vi "Local Setup Config.vi"(0 "KeyName":string, 1 "Local Setup Param":T1, 2 "Config File Directory":path, 5 "KeyValue":string, 9 "Last VI":string, 11 "error in":errorcluster) -> (6 "KeyValues":string[](array[string]), 8 "KeyNames":string[](array[string]), 10 "LastVIs":string[](array[string]), 15 "error out":errorcluster)   [LabVIEW 2014, in "Raspberry Pi Compatible Compiler for LabVIEW.lvlib"]
doc: "Functional Global for reading/writing configuration settings."
uses:
  Raspberry Pi Compatible Compiler for LabVIEW.lvlib
  Custom Controls/Local Setup Parameters.ctl
  <vilib>/Utility/config.llb/Write Key (String).vi
  <vilib>/Utility/config.llb/Read Key (String).vi
  <vilib>/Utility/config.llb/NI_LVConfig.lvlib
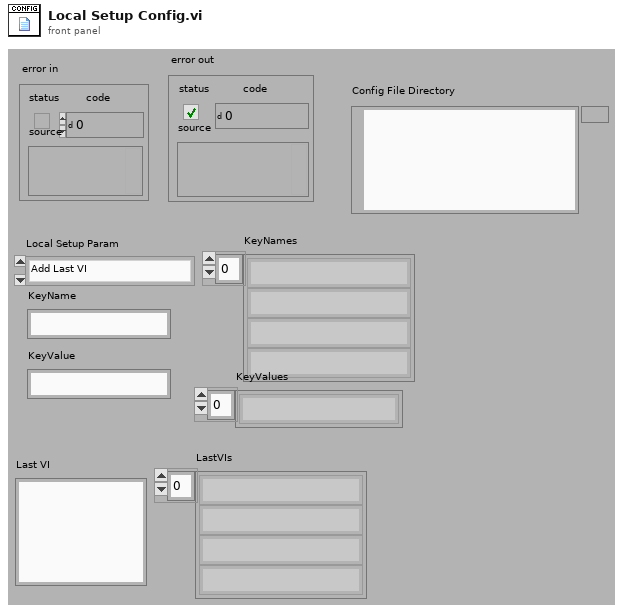
[diagram p1: front panel]
types:
  T1 = typedef "Raspberry Pi Compatible Compiler for LabVIEW.lvlib/Local Setup Parameters.ctl" = enum16{"Add Last VI", "Read Last VI", "Add Board IP", "Remove Board IP", "Read All Board IP", "Add Runtime Version", "Read Runtime Version", "Add Package Version", "Read Package Version", "Add VIPCheck Time", "Read VIPCheck Time"}
  T2 = typedef "NI_LVConfig.lvlib/Config Data RefNum.ctl" = refnum<k1>
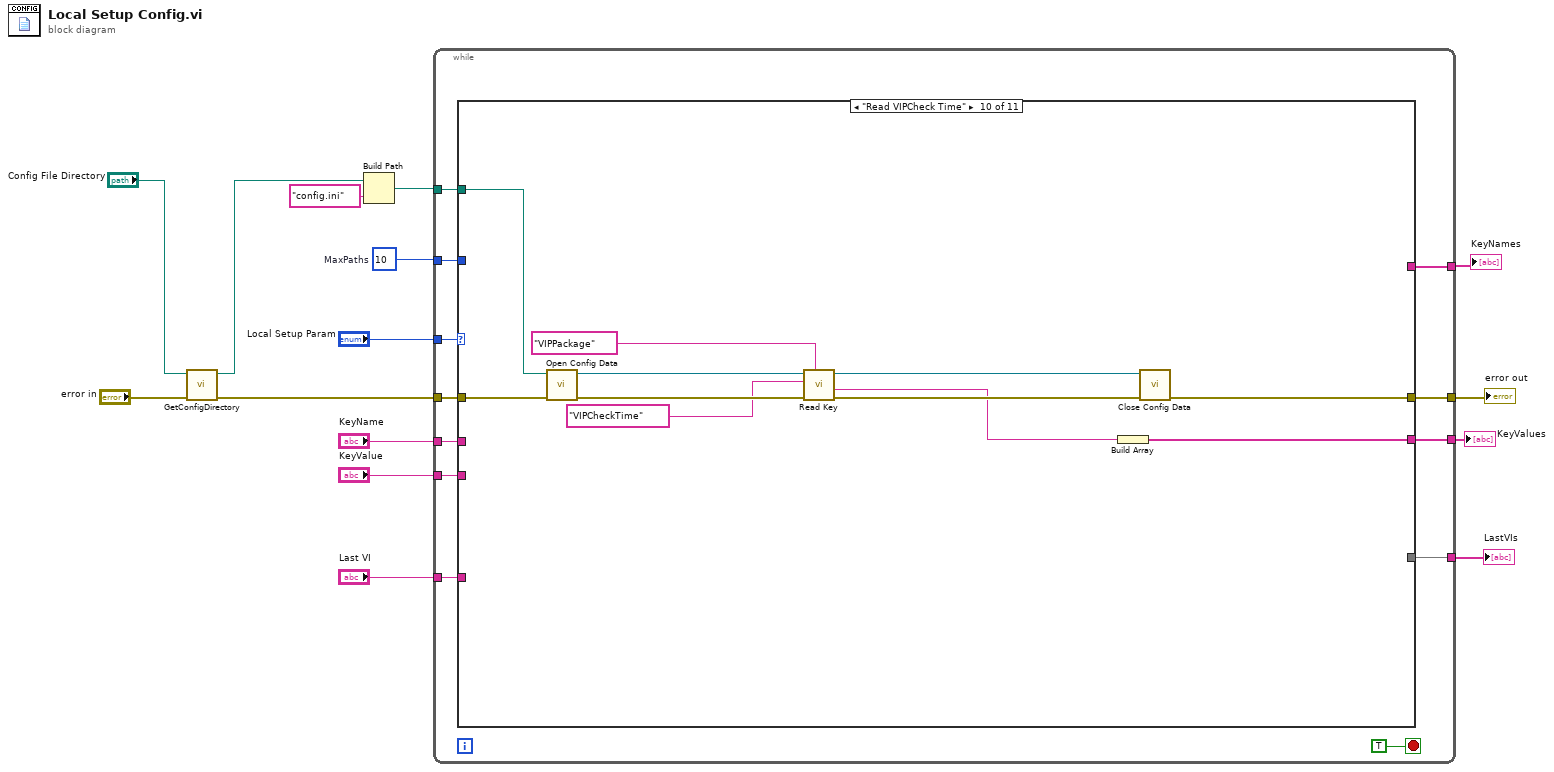
[diagram p0: block diagram]
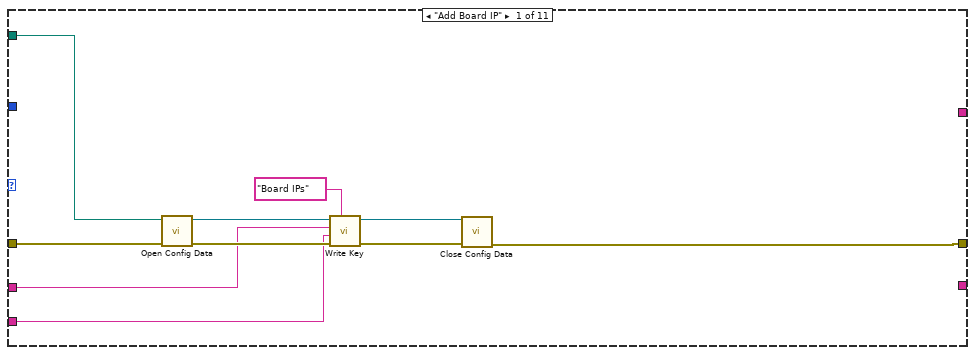
[diagram p2: hidden frame]
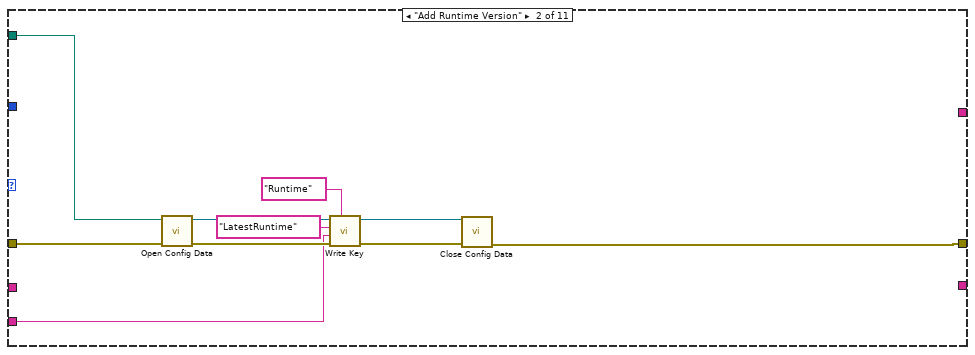
[diagram p3: hidden frame]
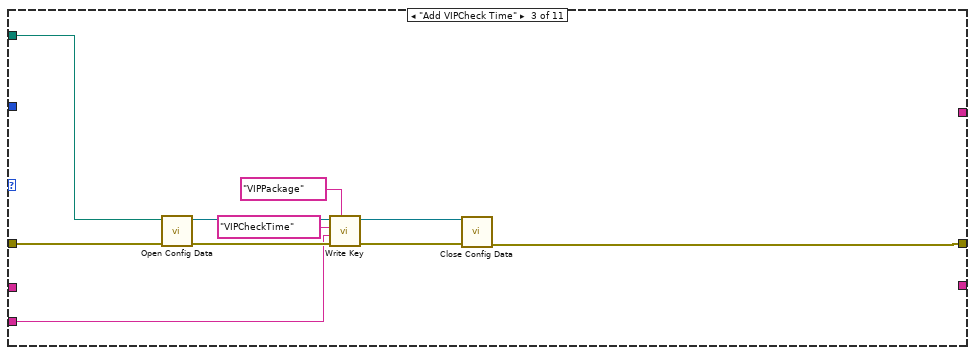
[diagram p4: hidden frame]
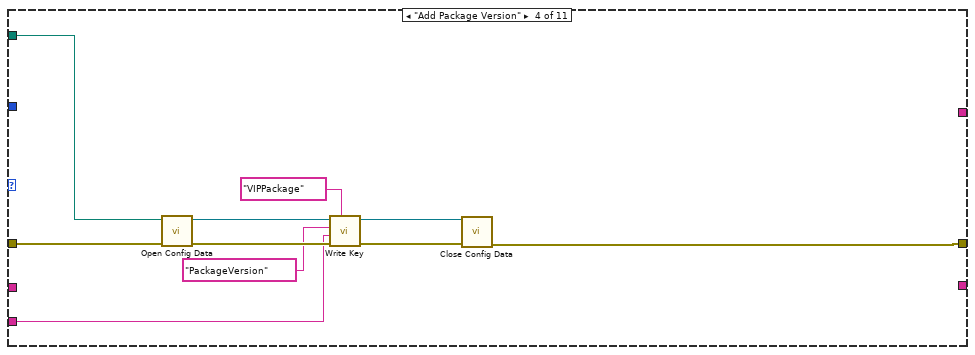
[diagram p5: hidden frame]
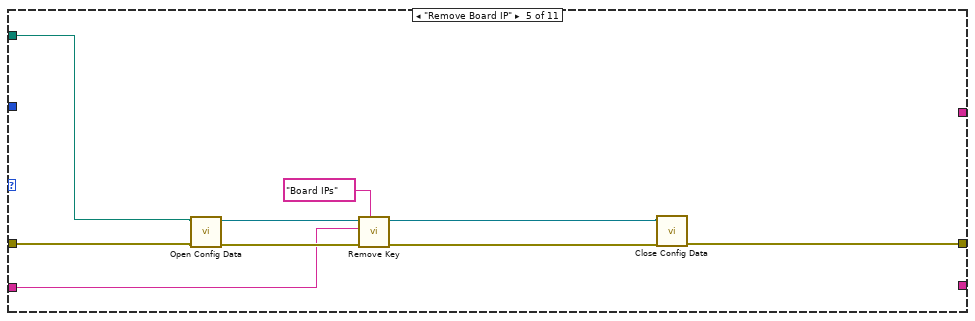
[diagram p6: hidden frame]
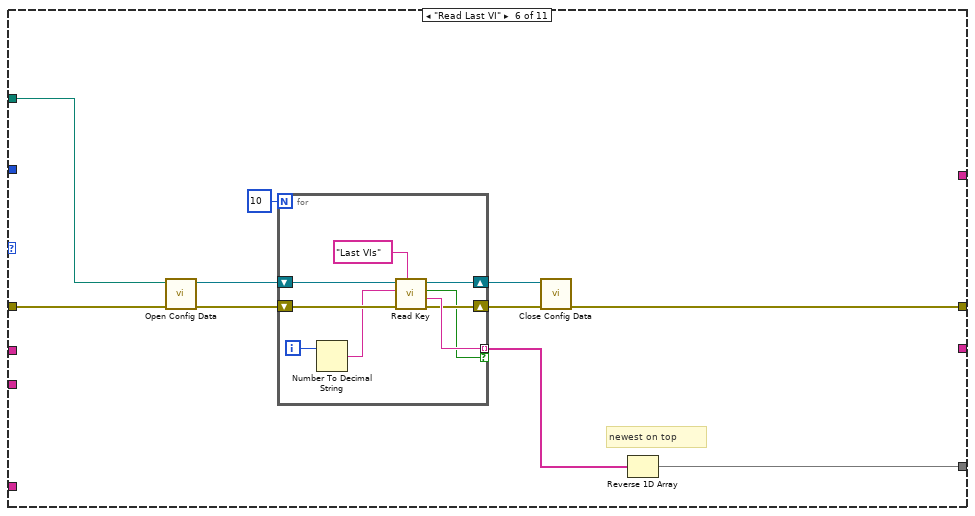
[diagram p7: hidden frame]
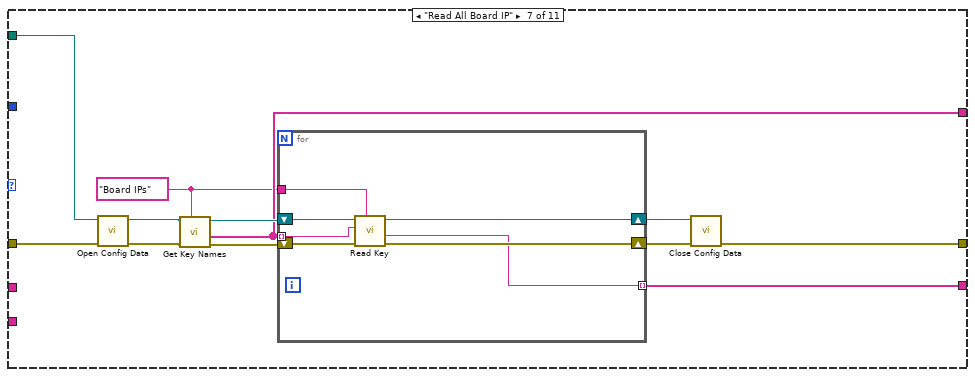
[diagram p8: hidden frame]
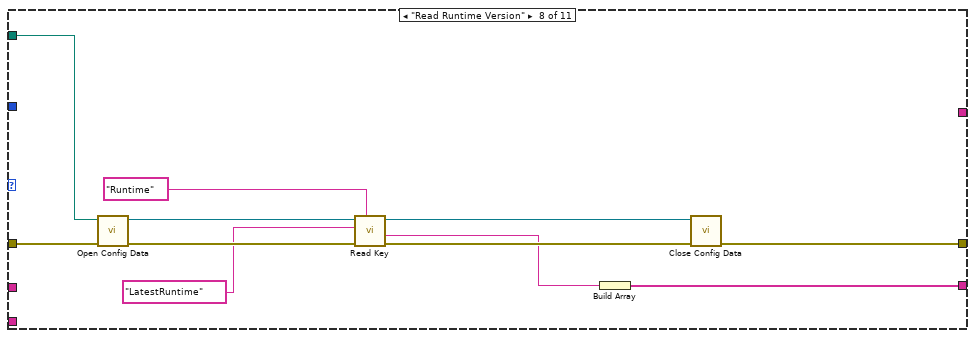
[diagram p9: hidden frame]
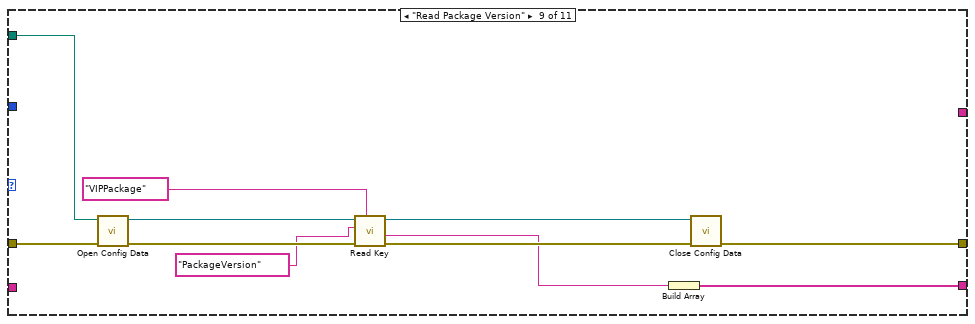
[diagram p10: hidden frame]
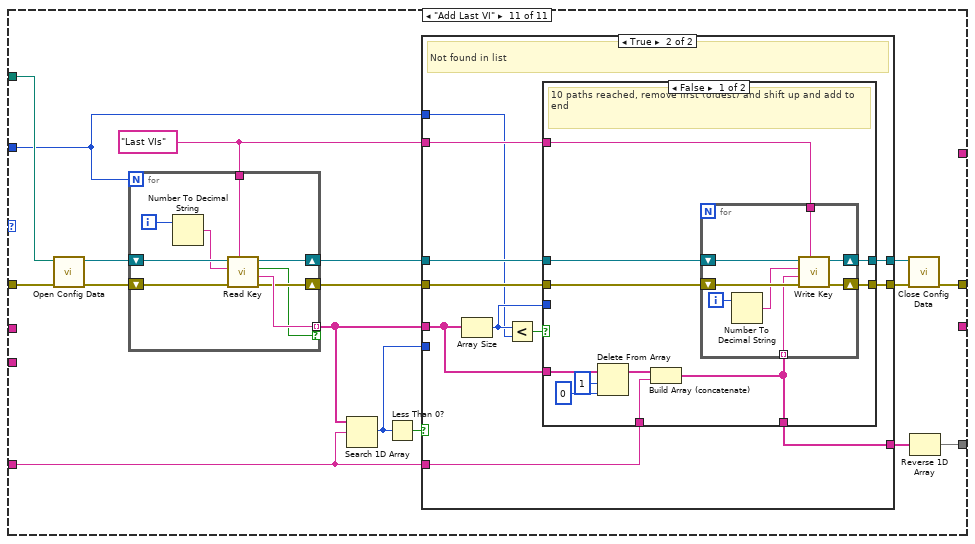
[diagram p11: hidden frame]
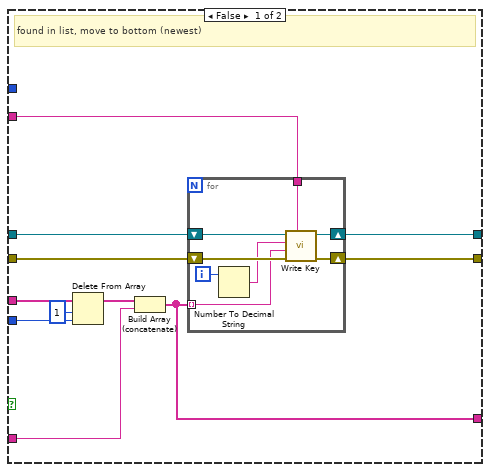
[diagram p12: hidden frame]
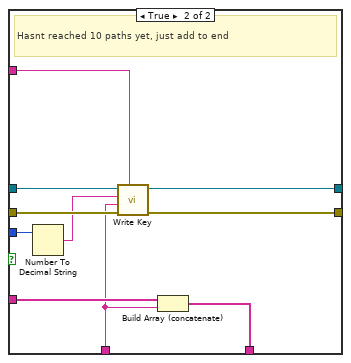
[diagram p13: hidden frame]
diagram:
  w8 = 10  # MaxPaths
  n1 = call "GetConfigDirectory.vi"("error in"="error in", "Config File Directory"="Config File Directory") -> ("error out"=w1:errorcluster, "config file directory out"=w4:path)  [unwired: 8 in]
  n2 = Build Path(base path=w4, name or relative path="config.ini") -> (appended path=w13:path)
  n3 = while {
    tunnel: "Local Setup Param" -> [w26]
    tunnel: w1 -> [w25]
    tunnel: "KeyName" -> [w24]
    tunnel: w13 -> [w23]
    tunnel: "KeyValue" -> [w22]
    tunnel: [w21] -> w11
    tunnel: [w20] -> w10
    tunnel: "Last VI" -> [w19]
    tunnel: w8 -> [w18]
    tunnel: [w17] -> w6
    tunnel: [w16] -> w5
    stop <- TRUE stop-if-true
    n4 = case shown="\"Read VIPCheck Time\"" w26 {
      tunnel: w25 -> [w35 w45 w55 w65 w73 w86 w107 w125 w136 w147 w164]
      tunnel: w24 -> [w33 _ _ _ w71 _ _ _ _ _ _]
      tunnel: w23 -> [w34 w44 w54 w64 w72 w85 w106 w124 w135 w146 w163]
      tunnel: w22 -> [w28 w39 w49 w59 _ _ _ _ _ _ _]
      tunnel: [w30 w41 w51 w61 w76 w82 w105 w123 w134 w145 w160] -> w21
      tunnel: [_ _ _ _ _ w77 _ _ _ _ w148] -> w20
      tunnel: w19 -> [_ _ _ _ _ _ _ _ _ _ w152]
      tunnel: w18 -> [_ _ _ _ _ _ _ _ _ _ w154]
      tunnel: [_ _ _ _ _ _ w98 _ _ _ _] -> w17
      tunnel: [_ _ _ _ _ _ w97 w118 w126 w138 _] -> w16
      frame "Add Board IP" {
        n5 = call <vilib>:"Open Config Data.vi"("error in (no error)"=w35, "configuration file path"=w34) -> ("error out"=w37:errorcluster, "refnum"=w36:T2)  [unwired: 7 in, 1 out]
        n6 = call-poly <vilib>:"Write Key.vi"("section"="Board IPs", "error in (no error)"=w37, "value"=w28, "key"=w33, "refnum"=w36) -> ("error out"=w31:errorcluster, "refnum out"=w32:T2)  [unwired: 4 in, 1 out]
        n7 = call <vilib>:"Close Config Data.vi"("error in (no error)"=w31, "refnum"=w32) -> ("error out"=w30:errorcluster)  [unwired: 8 in, 1 out]
      }
      frame "Add Runtime Version" {
        n8 = call <vilib>:"Open Config Data.vi"("error in (no error)"=w45, "configuration file path"=w44) -> ("error out"=w47:errorcluster, "refnum"=w46:T2)  [unwired: 7 in, 1 out]
        n9 = call-poly <vilib>:"Write Key.vi"("section"="Runtime", "error in (no error)"=w47, "value"=w39, "key"="LatestRuntime", "refnum"=w46) -> ("error out"=w42:errorcluster, "refnum out"=w43:T2)  [unwired: 4 in, 1 out]
        n10 = call <vilib>:"Close Config Data.vi"("error in (no error)"=w42, "refnum"=w43) -> ("error out"=w41:errorcluster)  [unwired: 8 in, 1 out]
      }
      frame "Add VIPCheck Time" {
        n11 = call <vilib>:"Open Config Data.vi"("error in (no error)"=w55, "configuration file path"=w54) -> ("error out"=w57:errorcluster, "refnum"=w56:T2)  [unwired: 7 in, 1 out]
        n12 = call-poly <vilib>:"Write Key.vi"("section"="VIPPackage", "error in (no error)"=w57, "value"=w49, "key"="VIPCheckTime", "refnum"=w56) -> ("error out"=w52:errorcluster, "refnum out"=w53:T2)  [unwired: 4 in, 1 out]
        n13 = call <vilib>:"Close Config Data.vi"("error in (no error)"=w52, "refnum"=w53) -> ("error out"=w51:errorcluster)  [unwired: 8 in, 1 out]
      }
      frame "Add Package Version" {
        n14 = call <vilib>:"Open Config Data.vi"("error in (no error)"=w65, "configuration file path"=w64) -> ("error out"=w67:errorcluster, "refnum"=w66:T2)  [unwired: 7 in, 1 out]
        n15 = call-poly <vilib>:"Write Key.vi"("section"="VIPPackage", "error in (no error)"=w67, "value"=w59, "key"="PackageVersion" ("section"), "refnum"=w66) -> ("error out"=w62:errorcluster, "refnum out"=w63:T2)  [unwired: 4 in, 1 out]
        n16 = call <vilib>:"Close Config Data.vi"("error in (no error)"=w62, "refnum"=w63) -> ("error out"=w61:errorcluster)  [unwired: 8 in, 1 out]
      }
      frame "Remove Board IP" {
        n17 = call <vilib>:"Open Config Data.vi"("error in (no error)"=w73, "configuration file path"=w72) -> ("error out"=w75:errorcluster, "refnum"=w74:T2)  [unwired: 7 in, 1 out]
        n18 = call <vilib>:"Remove Key.vi"("section"="Board IPs", "error in (no error)"=w75, "key"=w71, "refnum"=w74) -> ("error out"=w69:errorcluster, "refnum out"=w68:T2)  [unwired: 5 in, 1 out]
        n19 = call <vilib>:"Close Config Data.vi"("error in (no error)"=w69, "refnum"=w68) -> ("error out"=w76:errorcluster)  [unwired: 8 in, 1 out]
      }
      frame "Read Last VI" {
        # "newest on top"
        n20 = call <vilib>:"Open Config Data.vi"("error in (no error)"=w86, "configuration file path"=w85) -> ("error out"=w84:errorcluster, "refnum"=w83:T2)  [unwired: 7 in, 1 out]
        n21 = for {
          N: 10 -> [_]
          tunnel: [w92] -> w78 mode=indexing if=w87
          shift-right: [w91] -> w81
          shift-left: w84 -> [w95]
          shift-right: [w90] -> w80
          shift-left: w83 -> [w94]
          i -> [w89]
          n22 = Number To Decimal String(number=w89) -> (decimal integer string=w88:string)  [unwired: 1 in]
          n23 = call-poly <vilib>:"Read Key.vi"("section"="Last VIs", "error in (no error)"=w95, "key"=w88, "refnum"=w94) -> ("error out"=w91:errorcluster, "value"=w92:string, "found?"=w87:bool, "refnum out"=w90:T2)  [unwired: 4 in]
        }
        n24 = call <vilib>:"Close Config Data.vi"("error in (no error)"=w81, "refnum"=w80) -> ("error out"=w82:errorcluster)  [unwired: 8 in, 1 out]
        n25 = Reverse 1D Array(array=w78) -> (reversed array=w77:string[])
      }
      frame "Read All Board IP" {
        w96 = "Board IPs" ("section")
        n26 = call <vilib>:"Open Config Data.vi"("error in (no error)"=w107, "configuration file path"=w106) -> ("error out"=w101:errorcluster, "refnum"=w102:T2)  [unwired: 7 in, 1 out]
        n27 = call <vilib>:"Get Key Names.vi"("section"=w96, "error in (no error)"=w101, "refnum"=w102) -> ("error out"=w99:errorcluster, "key names"=w98:string[], "refnum out"=w100:T2)  [unwired: 5 in, 1 out]
        n28 = for {
          tunnel: [w110] -> w97 mode=indexing
          shift-right: [w112] -> w104
          shift-left: w99 -> [w114]
          shift-right: [w111] -> w103
          shift-left: w100 -> [w113]
          tunnel: w98 -> [w109] mode=indexing
          tunnel: w96 -> [w108]
          n29 = call-poly <vilib>:"Read Key.vi"("section"=w108, "error in (no error)"=w114, "key"=w109, "refnum"=w113) -> ("error out"=w112:errorcluster, "value"=w110:string, "refnum out"=w111:T2)  [unwired: 4 in, 1 out]
        }
        n30 = call <vilib>:"Close Config Data.vi"("error in (no error)"=w104, "refnum"=w103) -> ("error out"=w105:errorcluster)  [unwired: 8 in, 1 out]
      }
      frame "Read Runtime Version" {
        n31 = call <vilib>:"Open Config Data.vi"("error in (no error)"=w125, "configuration file path"=w124) -> ("error out"=w116:errorcluster, "refnum"=w117:T2)  [unwired: 7 in, 1 out]
        n32 = call-poly <vilib>:"Read Key.vi"("section"="Runtime", "error in (no error)"=w116, "key"="LatestRuntime", "refnum"=w117) -> ("error out"=w122:errorcluster, "value"=w120:string, "refnum out"=w121:T2)  [unwired: 4 in, 1 out]
        n33 = Build Array(w120) -> (w118:string[])
        n34 = call <vilib>:"Close Config Data.vi"("error in (no error)"=w122, "refnum"=w121) -> ("error out"=w123:errorcluster)  [unwired: 8 in, 1 out]
      }
      frame "Read Package Version" {
        n35 = call <vilib>:"Open Config Data.vi"("error in (no error)"=w136, "configuration file path"=w135) -> ("error out"=w130:errorcluster, "refnum"=w129:T2)  [unwired: 7 in, 1 out]
        n36 = call-poly <vilib>:"Read Key.vi"("section"="VIPPackage", "error in (no error)"=w130, "key"="PackageVersion" ("section"), "refnum"=w129) -> ("error out"=w133:errorcluster, "value"=w127:string, "refnum out"=w132:T2)  [unwired: 4 in, 1 out]
        n37 = Build Array(w127) -> (w126:string[])
        n38 = call <vilib>:"Close Config Data.vi"("error in (no error)"=w133, "refnum"=w132) -> ("error out"=w134:errorcluster)  [unwired: 8 in, 1 out]
      }
      frame "Read VIPCheck Time" {
        n39 = call <vilib>:"Open Config Data.vi"("error in (no error)"=w147, "configuration file path"=w146) -> ("error out"=w141:errorcluster, "refnum"=w140:T2)  [unwired: 7 in, 1 out]
        n40 = call-poly <vilib>:"Read Key.vi"("section"="VIPPackage", "error in (no error)"=w141, "key"="VIPCheckTime", "refnum"=w140) -> ("error out"=w144:errorcluster, "value"=w139:string, "refnum out"=w143:T2)  [unwired: 4 in, 1 out]
        n41 = Build Array(w139) -> (w138:string[])
        n42 = call <vilib>:"Close Config Data.vi"("error in (no error)"=w144, "refnum"=w143) -> ("error out"=w145:errorcluster)  [unwired: 8 in, 1 out]
      }
      frame "Add Last VI" {
        w157 = "Last VIs" ("section")
        n43 = call <vilib>:"Open Config Data.vi"("error in (no error)"=w164, "configuration file path"=w163) -> ("error out"=w162:errorcluster, "refnum"=w161:T2)  [unwired: 7 in, 1 out]
        n44 = for {
          N: w154 -> [_]
          tunnel: [w230] -> w153 mode=indexing if=w225
          shift-right: [w229] -> w159
          shift-left: w162 -> [w232]
          shift-right: [w228] -> w158
          shift-left: w161 -> [w231]
          tunnel: w157 -> [w224]
          i -> [w227]
          n45 = Number To Decimal String(number=w227) -> (decimal integer string=w226:string)  [unwired: 1 in]
          n46 = call-poly <vilib>:"Read Key.vi"("section"=w224, "error in (no error)"=w232, "key"=w226, "refnum"=w231) -> ("error out"=w229:errorcluster, "value"=w230:string, "found?"=w225:bool, "refnum out"=w228:T2)  [unwired: 4 in]
        }
        n47 = Search 1D Array(1D array=w153, element=w152) -> (index of element=w150:i32)  [unwired: 1 in]
        n48 = Less Than 0?(x=w150) -> (x < 0?=w151:bool)
        n49 = case shown="True" w151 {
          tunnel: w159 -> [w170 w193]
          tunnel: w158 -> [w169 w192]
          tunnel: w157 -> [w166 w191]
          tunnel: [w167 w189] -> w156
          tunnel: [w168 w188] -> w155
          tunnel: w154 -> [_ w187]
          tunnel: w153 -> [w175 w185]
          tunnel: w152 -> [w171 w186]
          tunnel: w150 -> [w174 _]
          tunnel: [w165 w184] -> w149
          frame False {
            # "found in list, move to bottom (newest)"
            n50 = Delete From Array(array=w175, length=1, index=w174) -> (array with subset deleted=w172:string[])  [unwired: 1 out]
            n51 = Build Array (concatenate)(w172, w171) -> (w165:string[])
            n52 = for {
              shift-right: [w181] -> w168
              shift-left: w169 -> [w182]
              shift-right: [w180] -> w167
              shift-left: w170 -> [w183]
              tunnel: w166 -> [w179]
              tunnel: w165 -> [w176] mode=indexing
              i -> [w178]
              n53 = Number To Decimal String(number=w178) -> (decimal integer string=w177:string)  [unwired: 1 in]
              n54 = call-poly <vilib>:"Write Key.vi"("section"=w179, "error in (no error)"=w183, "value"=w176, "key"=w177, "refnum"=w182) -> ("error out"=w180:errorcluster, "refnum out"=w181:T2)  [unwired: 4 in, 1 out]
            }
          }
          frame True {
            # "Not found in list"
            n55 = Array Size(array=w185) -> (size(s)=w190:i32)
            n56 = Less?(x=w190, y=w187) -> (x < y?=w194:bool)
            n57 = case shown="False" w194 {
              tunnel: w193 -> [w199 w223]
              tunnel: w192 -> [w200 w221]
              tunnel: w191 -> [w196 w222]
              tunnel: w190 -> [_ w220]
              tunnel: w186 -> [w201 w215]
              tunnel: [w197 w218] -> w189
              tunnel: [w198 w217] -> w188
              tunnel: w185 -> [w204 w216]
              tunnel: [w195 w214] -> w184
              frame False {
                # "10 paths reached, remove first (oldest) and shift up and add to end"
                n58 = Delete From Array(array=w204, length=1, index=0) -> (array with subset deleted=w202:string[])  [unwired: 1 out]
                n59 = Build Array (concatenate)(w202, w201) -> (w195:string[])
                n60 = for {
                  shift-right: [w211] -> w198
                  shift-left: w200 -> [w212]
                  shift-right: [w210] -> w197
                  shift-left: w199 -> [w213]
                  tunnel: w195 -> [w207] mode=indexing
                  tunnel: w196 -> [w206]
                  i -> [w209]
                  n61 = Number To Decimal String(number=w209) -> (decimal integer string=w208:string)  [unwired: 1 in]
                  n62 = call-poly <vilib>:"Write Key.vi"("section"=w206, "error in (no error)"=w213, "value"=w207, "key"=w208, "refnum"=w212) -> ("error out"=w210:errorcluster, "refnum out"=w211:T2)  [unwired: 4 in, 1 out]
                }
              }
              frame True {
                # "Hasnt reached 10 paths yet, just add to end"
                n63 = Number To Decimal String(number=w220) -> (decimal integer string=w219:string)  [unwired: 1 in]
                n64 = call-poly <vilib>:"Write Key.vi"("section"=w222, "error in (no error)"=w223, "value"=w215, "key"=w219, "refnum"=w221) -> ("error out"=w218:errorcluster, "refnum out"=w217:T2)  [unwired: 4 in, 1 out]
                n65 = Build Array (concatenate)(w216, w215) -> (w214:string[])
              }
            }
          }
        }
        n66 = call <vilib>:"Close Config Data.vi"("error in (no error)"=w156, "refnum"=w155) -> ("error out"=w160:errorcluster)  [unwired: 8 in, 1 out]
        n67 = Reverse 1D Array(array=w149) -> (reversed array=w148:string[])
      }
    }
  }
  "error out" <- w11
  "LastVIs" <- w10
  "KeyNames" <- w6
  "KeyValues" <- w5
